vi "Solenoid.vi"   [LabVIEW 2012]
uses:
  <vilib>/Rock Robotics/WPI/Solenoid/WPI_SolenoidValue.ctl
  <vilib>/Rock Robotics/WPI/Compressor/WPI_CompressorGetSetRefNum.vi
  Robot Global Data.vi
  <vilib>/Rock Robotics/WPI/Solenoid/WPI_SolenoidSetEnum.vi
types:
  T1 = typedef "WPI_SolenoidDevRef.ctl" = cluster{"DevStatus":errorcluster, "Solenoid Module":T2, "Forward Solenoid Channel":T3, "Reverse Solenoid Channel":T3}
  T2 = typedef "FPGA_TypedefSolenoidModule.ctl" = enum16{"Solenoid Module 1", "Solenoid Module 2"}
  T3 = typedef "WPI_SolenoidChannel.ctl" = enum8{"Solenoid 1", "Solenoid 2", "Solenoid 3", "Solenoid 4", "Solenoid 5", "Solenoid 6", "Solenoid 7", "Solenoid 8", "Invalid"}
  T4 = typedef "WPI_CompressorDevRef.ctl" = cluster{"DevStatus":errorcluster, "DigitalInputDevRef":T5, "RelayDevRef":T8}
  T5 = typedef "WPI_DigitalInputDevRef.ctl" = cluster{"DevStatus":errorcluster, "DIO Channel":T6, "Digital Module":T7}
  T6 = typedef "FPGA_DIOChannel.ctl" = enum8{"DIO 1", "DIO 2", "DIO 3", "DIO 4", "DIO 5", "DIO 6", "DIO 7", "DIO 8", "DIO 9", "DIO 10", "DIO 11", "DIO 12", "DIO 13", "DIO 14", "Invalid"}
  T7 = typedef "FPGA_TypedefDigitalModule.ctl" = enum16{"Digital Module 1", "Digital Module 2"}
  T8 = typedef "WPI_RelayDevRef.ctl" = cluster{"DevStatus":errorcluster, "Relay Channel":T9, "Digital Module":T7, "Relay Direction":T10}
  T9 = typedef "FPGA_DIORelayChannel.ctl" = enum8{"Relay 1", "Relay 2", "Relay 3", "Relay 4", "Relay 5", "Relay 6", "Relay 7", "Relay 8", "Invalid"}
  T10 = typedef "WPI_RelayDirection.ctl" = enum16{"Both directions", "Forward only", "Reverse only"}
  T11 = typedef "WPI_SolenoidValue.ctl" = enum16{"Off", "On", "Forward", "Reverse"}
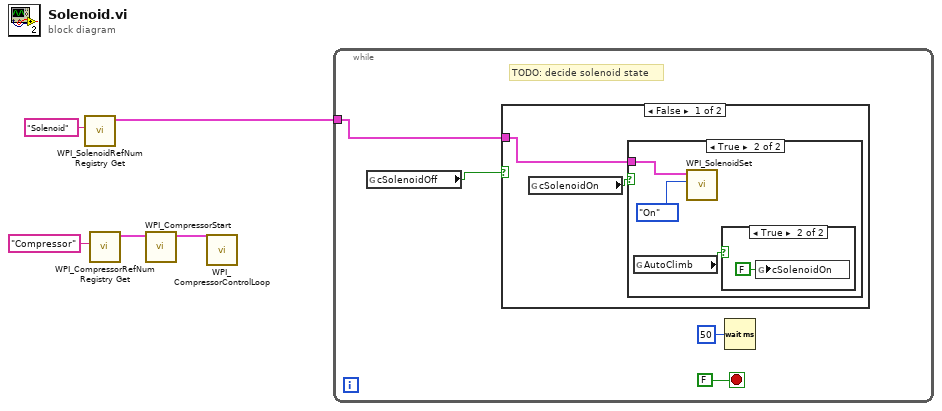
[diagram p0: block diagram]
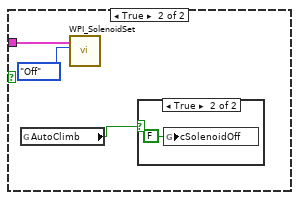
[diagram p4: hidden frame]
diagram:
  n1 = call <vilib>:"WPI_SolenoidRefNum Registry Get.vi"("refnum name"="Solenoid") -> ("SolenoidDevRef"=w1:T1)  [unwired: 9 in, 1 out]
  n2 = call <vilib>:"WPI_CompressorRefNum Registry Get.vi"("refnum name"="Compressor") -> ("CompressorDevRef"=w5:T4)  [unwired: 9 in, 1 out]
  n3 = call <vilib>:"WPI_CompressorStart.vi"("CompressorDevRef"=w5) -> ("CompressorDevRef"=w3:T4)  [unwired: 9 in, 1 out]
  n4 = call <vilib>:"WPI_CompressorControlLoop.vi"("CompressorDevRef"=w3) -> ()  [unwired: 11 in]
  n5 = while {
    tunnel: w1 -> [w7]
    stop <- FALSE stop-if-true
    # "TODO: decide solenoid state"
    n6 = global read "Robot Global Data.vi" "cSolenoidOff"() -> (w8:bool)
    n7 = case shown="False" w8 {
      tunnel: w7 -> [w10 w18]
      frame False {
        n8 = global read "Robot Global Data.vi" "cSolenoidOn"() -> (w11:bool)
        n9 = case shown="True" w11 {
          tunnel: w10 -> [_ w14]
          frame False {
          }
          frame True {
            n10 = global read "Robot Global Data.vi" "AutoClimb"() -> (w12:bool)
            n11 = call-poly <vilib>:"WPI_SolenoidSet.vi"("Value"=WPI_SolenoidValue."On", "SolenoidDevRef"=w14) -> ()  [unwired: 8 in, 2 out]
            n12 = case shown="True" w12 {
              frame False {
              }
              frame True {
                n13 = global write "Robot Global Data.vi" "cSolenoidOn"(FALSE ("cSolenoidOn")) -> ()
              }
            }
          }
        }
      }
      frame True {
        n14 = global read "Robot Global Data.vi" "AutoClimb"() -> (w16:bool)
        n15 = call-poly <vilib>:"WPI_SolenoidSet.vi"("Value"=WPI_SolenoidValue."Off", "SolenoidDevRef"=w18) -> ()  [unwired: 8 in, 2 out]
        n16 = case shown="True" w16 {
          frame False {
          }
          frame True {
            n17 = global write "Robot Global Data.vi" "cSolenoidOff"(FALSE ("cSolenoidOff")) -> ()
          }
        }
      }
    }
    n18 = Wait (ms)(milliseconds to wait=u32 50) -> ()  [unwired: 1 out]
  }
